vi "output.vi"() -> (1 "ok?":bool, 2 "txt?excel":string, 3 "path":path)   [LabVIEW 2011]
panel:
  in  "cancel":bool
  in  "ok":bool
  in  "文件名称":string
  in  "存放路径":path
  in  "格式":enum32{"文本文件", "EXCEL文件"}(radio)
  # "选项"
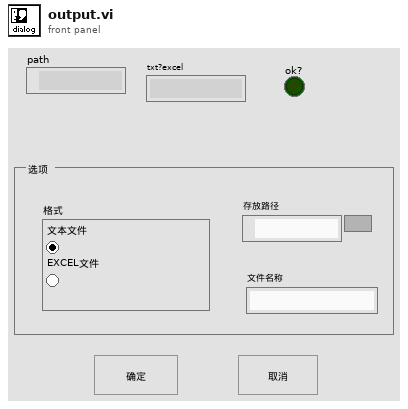
[diagram p1: front panel]
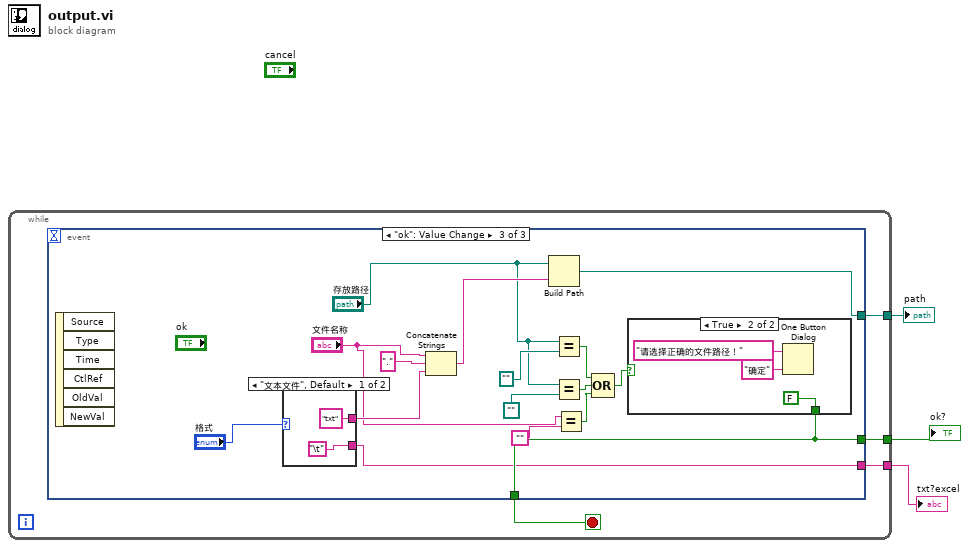
[diagram p0: block diagram]
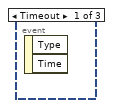
[diagram p2: hidden frame]
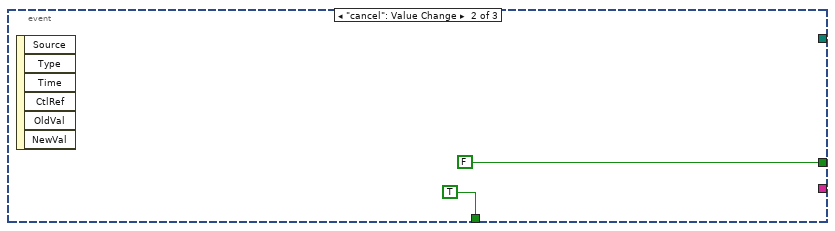
[diagram p3: hidden frame]
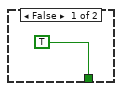
[diagram p4: hidden frame]
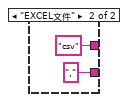
[diagram p5: hidden frame]
diagram:
  n1 = while {
    tunnel: [w6] -> w2
    tunnel: [w5] -> w1
    tunnel: [w4] -> w3
    stop <- w7 stop-if-true
    n2 = event shown="[2] \"ok\": Value Change" {
      selector: _ -> [_ _ _]
      dyn-events: _ -> [_ _ _]
      timeout: _ -> [_ _ _]
      tunnel: [_ TRUE w18] -> w7
      tunnel: [_ FALSE w18] -> w6
      tunnel: [_ _ w19] -> w5
      tunnel: [_ _ w10] -> w4
      event Timeout {
        n3 = event-data() -> ()  [unwired: 3 out]
      }
      event "cancel": Value Change {
        n4 = event-data() -> ()  [unwired: 7 out]
      }
      event "ok": Value Change {
        n5 = event-data() -> ()  [unwired: 7 out]
        n6 = case shown="\"文本文件\", Default" "格式" {
          tunnel: ["txt" "csv"] -> w22
          tunnel: ["\t" ","] -> w10
          frame "文本文件", Default {
          }
          frame "EXCEL文件" {
          }
        }
        n7 = Concatenate Strings("文件名称", "." ("string"), w22) -> (w25:string)
        n8 = Build Path(base path="存放路径", name or relative path=w25) -> (appended path=w19:path)
        n9 = Equal?(x="存放路径", y=path "") -> (x = y?=w14:bool)
        n10 = Equal?(x="存放路径", y=path "") -> (x = y?=w13:bool)
        n11 = Equal?(x="文件名称", y="") -> (x = y?=w12:bool)
        n12 = Compound Arithmetic op=OR(w14, w13, w12) -> (w11:bool)
        n13 = case shown="True" w11 {
          tunnel: [TRUE FALSE] -> w18
          frame False {
          }
          frame True {
            n14 = One Button Dialog(message="请选择正确的文件路径！", button name ("OK")="确定") -> ()  [unwired: 1 out]
          }
        }
      }
    }
  }
  "txt?excel" <- w3
  "ok?" <- w2
  "path" <- w1
